vi "Upload Board.vi"(8 "error in (no error)":errorcluster, 11 "Board_Game in":refnum<class "Board_Game.lvclass">) -> (0 "error out":errorcluster, 3 "Board_Game out":refnum<class "Board_Game.lvclass">)   [LabVIEW 2021, in "Board_Game.lvclass"]
uses:
  Board_Game.lvclass
  Board_Game.lvclass/Board_Game.ctl
  SnakeGame/Snake.lvclass
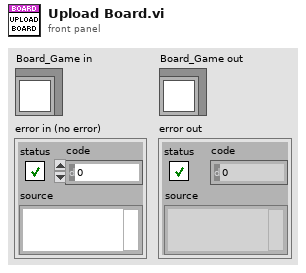
[diagram p1: front panel]
types:
  T1 = typedef "Position.ctl" = cluster{"X":u32, "Y":u32}
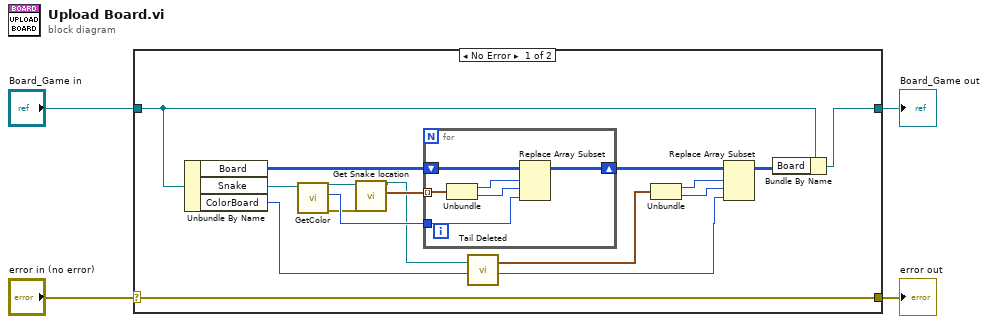
[diagram p0: block diagram]
diagram:
  n1 = case shown="No Error" "error in (no error)" {
    selector: "error in (no error)" -> [w20 w28]
    tunnel: [w20 w28] -> w3
    tunnel: [w18 w27] -> w1
    tunnel: "Board_Game in" -> [w19 w27]
    frame No Error {
      n2 = Unbundle By Name(w19) -> ("Board"=w13:u32[][], "Snake"=w16:refnum<class "Snake.lvclass">, "ColorBoard"=w7:u32)
      n3 = call-dynamic "GetColor.vi"("SnakeGame in"=w16) -> ("error out"=w15:errorcluster, "Color"=w17:u32, "SnakeGame out"=w12:refnum<class "Snake.lvclass">)  [unwired: 8 in]
      n4 = call-dynamic "Get Snake location.vi"("error in (no error)"=w15, "Snake in"=w12) -> ("Snake location"=w14:T1[], "Snake out"=w6:refnum<class "Snake.lvclass">)  [unwired: 7 in, 1 out]
      n5 = for {
        tunnel: w17 -> [w24]
        tunnel: w14 -> [w23] mode=indexing
        shift-right: [w25] -> w9
        shift-left: w13 -> [w26]
        n6 = Unbundle(w23) -> ("X"=w22:u32, "Y"=w21:u32)
        n7 = Replace Array Subset "Replace Array Subset"(array=w26, new element=w24, index (row)=w22, index (col)=w21) -> (w25:u32[][])
      }
      n8 = call "Tail Deleted.vi"("Snake in"=w6) -> ("Tail deleted"=w5:T1)  [unwired: 2 in]
      n9 = Unbundle(w5) -> ("X"=w11:u32, "Y"=w10:u32)
      n10 = Replace Array Subset(array=w9, new element=w7, index (row)=w11, index (col)=w10) -> (w8:u32[][])
      n11 = Bundle By Name(cluster=w19, "Board"=w8) -> (w18:refnum<class "Board_Game.lvclass">)
    }
    frame Error {
    }
  }
  "error out" <- w3
  "Board_Game out" <- w1
